vi "Waveform_Append and Resize Unallocated.vi"(8 "Time Of Buffer (S)":dbl, 9 "Append":T1, 11 "Waveform":T1) -> (0 "Total Starting Offset Out":i32, 1 "End Point Out":i32, 2 "Start Pointer Out":i32, 3 "Waveform Out":T1, 5 "Reset Time Out":bool)   [LabVIEW 2015]
uses:
  Universal Controls/Waveform_Data.ctl
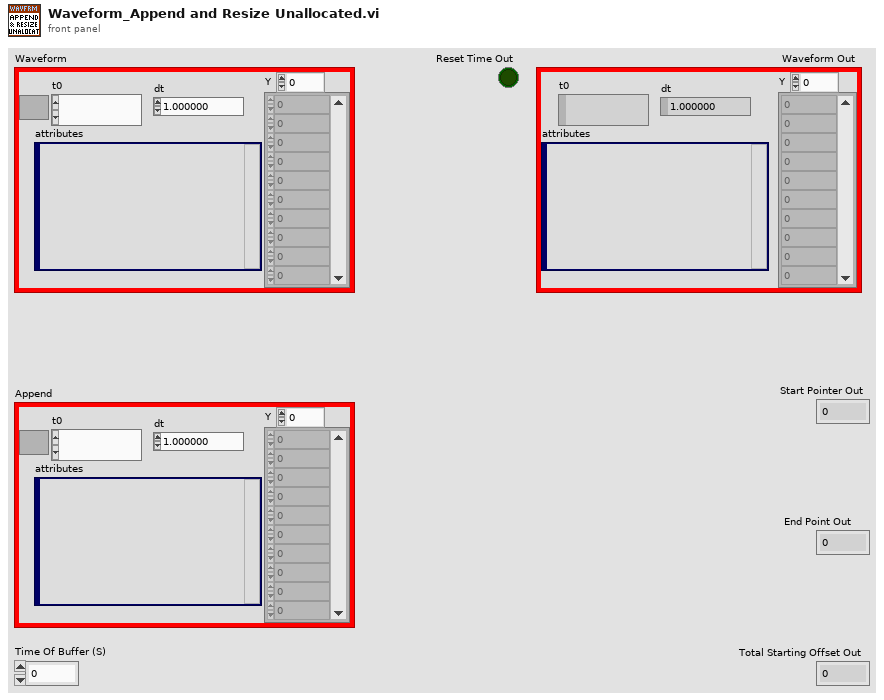
[diagram p1: front panel]
types:
  T1 = typedef "Waveform_Data.ctl" = waveform(dbl)
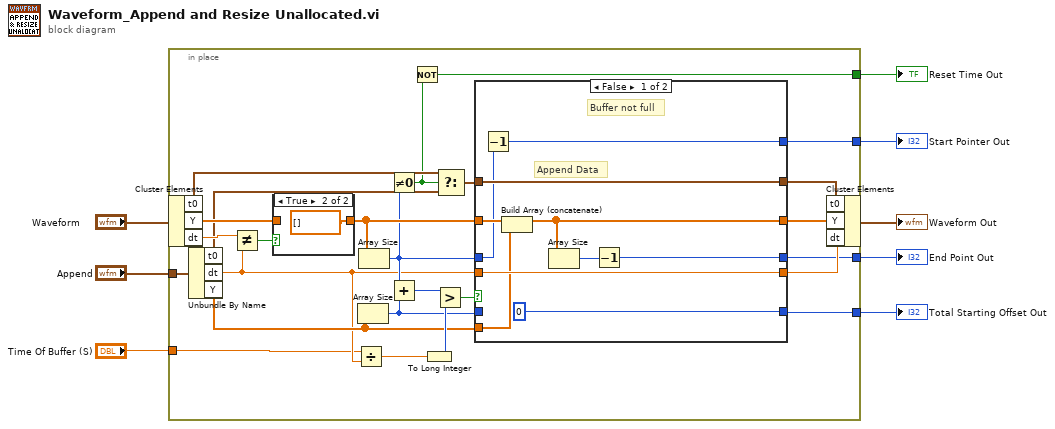
[diagram p0: block diagram]
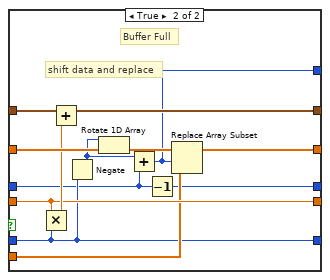
[diagram p2: hidden frame]
diagram:
  n1 = in-place {
    in-place-border: [w13] -> w2
    in-place-border: [w28] -> w1
    in-place-border: "Append" -> [w30]
    in-place-border: "Time Of Buffer (S)" -> [w9]
    in-place-border: [w23] -> w5
    in-place-border: [w20] -> w6
    n2 = in-place-cluster #1("Waveform") -> ("t0"=w33:timestamp, "Y"=w31:dbl[], "dt"=w24:dbl)
    n3 = Unbundle By Name(w30) -> ("t0"=w10:timestamp, "dt"=w11:dbl, "Y"=w17:dbl[])
    n4 = Not Equal?(x=w24, y=w11) -> (x != y?=w32:bool)
    n5 = case shown="True" w32 {
      tunnel: w31 -> [w57 _]
      tunnel: [w57 dbl[] [] ("Y")] -> w16
      frame False {
      }
      frame True {
      }
    }
    n6 = Divide(x=w9, y=w11) -> (x/y=w19:dbl)
    n7 = Array Size(array=w17) -> (size(s)=w14:i32)
    n8 = Array Size(array=w16) -> (size(s)=w12:i32)
    n9 = Not Equal To 0?(x=w12) -> (x != 0?=w21:bool)
    n10 = Add(x=w12, y=w14) -> (x+y=w15:i32)
    n11 = Not(x=w21) -> (.not. x?=w20:bool)
    n12 = To Long Integer(number=w19) -> (32bit integer=w18:i32)
    n13 = Greater?(x=w15, y=w18) -> (0:w29:bool)
    n14 = Select(t=w33, s=w21, f=w10) -> (s? t:f=w25:timestamp)
    n15 = case shown="False" w29 {
      tunnel: [w35 w48] -> w28
      tunnel: [w36 w44] -> w13
      tunnel: w16 -> [w40 w56]
      tunnel: [w38 w55] -> w27
      tunnel: w25 -> [w43 w53]
      tunnel: [w43 w52] -> w26
      tunnel: [0 w46] -> w23
      tunnel: w11 -> [w41 w51]
      tunnel: [w41 w51] -> w22
      tunnel: w17 -> [w39 w49]
      tunnel: w14 -> [_ w46]
      tunnel: w12 -> [w34 w45]
      frame False {
        # "Append Data"
        # "Buffer not full"
        n16 = Decrement(x=w34) -> (x-1=w35:i32)
        n17 = Build Array (concatenate)(w40, w39) -> (w38:dbl[])
        n18 = Array Size(array=w38) -> (size(s)=w37:i32)
        n19 = Decrement(x=w37) -> (x-1=w36:i32)
      }
      frame True {
        # "shift data and replace"
        # "Buffer Full"
        n20 = Multiply(x=w51, y=w46) -> (x*y=w54:dbl)
        n21 = Add(x=w53, y=w54) -> (x+y=w52:timestamp)
        n22 = Negate(x=w46) -> (-x=w47:i32)
        n23 = Rotate 1D Array(1:w56, 2:w47) -> (0:w50:dbl[])
        n24 = Add(x=w47, y=w45) -> (x+y=w48:i32)
        n25 = Decrement(x=w45) -> (x-1=w44:i32)
        n26 = Replace Array Subset(array=w50, new element=w49, index=w48) -> (w55:dbl[])
      }
    }
    n27 = in-place-cluster #1("t0"=w26, "Y"=w27, "dt"=w22) -> (→"Waveform Out":T1)
  }
  "Reset Time Out" <- w6
  "Total Starting Offset Out" <- w5
  "End Point Out" <- w2
  "Start Pointer Out" <- w1
